vi "nanocal -- nuclear schottky fit V4.vi"() -> ()   [LabVIEW 2020] (continued)
\"τ1\"-> 0.024702194699  , \"τS\"-> 0.049753720072  , \"τN\"-> 0.002517387539  , \"τC\"-> 0.001542602546  , \"κ0\"-> 0.000000001719  , \"mm1\"-> 0.000000000000  , \"mm2\"-> 0.000000000000  , \"mm3\"-> 0.000000000000  , \"T\"->  0.308000000000  , \"B\"-> 5.000000000000  , \"θ\"-> 90.000000000000  |>   , \n\"IDS0340_210904_RAW_cal__sam_\" ->   <| \"ζ\"->  0.049152938826  , \"τ1\"-> 0.019216107215  , \"τS\"-> 0.064101941953  , \"τN\"-> 0.003869712687  , \"τC\"-> 0.002203680801  , \"κ0\"-> 0.000000001878  , \"mm1\"-> 0.000000000000  , \"mm2\"-> 0.000000000000  , \"mm3\"-> 0.000000000000  , \"T\"->  0.308000000000  , \"B\"-> 5.000000000000  , \"θ\"-> 90.000000000000  |>   , \n\"IDS0341_210904_RAW_cal__ref_\" ->   <| \"ζ\"->  0.059616809183  , \"τ1\"-> 0.023939570797  , \"τS\"-> 0.042653632086  , \"τN\"-> 0.001786288241  , \"τC\"-> 0.001975926031  , \"κ0\"-> 0.000000002092  , \"mm1\"-> 0.000000000000  , \"mm2\"-> 0.000000000000  , \"mm3\"-> 0.000000000000  , \"T\"->  0.360000000000  , \"B\"-> 5.000000000000  , \"θ\"-> 90.000000000000  |>   , \n\"IDS0341_210904_RAW_cal__sam_\" ->   <| \"ζ\"->  0.036041476168  , \"τ1\"-> 0.019203470752  , \"τS\"-> 0.054931014880  , \"τN\"-> 0.002271152158  , \"τC\"-> 0.002720100083  , \"κ0\"-> 0.000000002280  , \"mm1\"-> 0.000000000000  , \"mm2\"-> 0.000000000000  , \"mm3\"-> 0.000000000000  , \"T\"->  0.360000000000  , \"B\"-> 5.000000000000  , \"θ\"-> 90.000000000000  |>   , \n\"IDS0342_210904_RAW_cal__ref_\" ->   <| \"ζ\"->  0.044217232361  , \"τ1\"-> 0.023574215500  , \"τS\"-> 0.035981580515  , \"τN\"-> 0.001074333911  , \"τC\"-> 0.002351862552  , \"κ0\"-> 0.000000002629  , \"mm1\"-> 0.000000000000  , \"mm2\"-> 0.000000000000  , \"mm3\"-> 0.000000000000  , \"T\"->  0.438000000000  , \"B\"-> 5.000000000000  , \"θ\"-> 90.000000000000  |>   , \n\"IDS0342_210904_RAW_cal__sam_\" ->   <| \"ζ\"->  0.027360242550  , \"τ1\"-> 0.019369895135  , \"τS\"-> 0.046063450687  , \"τN\"-> 0.001549427641  , \"τC\"-> 0.003313507267  , \"κ0\"-> 0.000000002850  , \"mm1\"-> 0.000000000000  , \"mm2\"-> 0.000000000000  , \"mm3\"-> 0.000000000000  , \"T\"->  0.438000000000  , \"B\"-> 5.000000000000  , \"θ\"-> 90.000000000000  |>   , \n\"IDS0343_210904_RAW_cal__ref_\" ->   <| \"ζ\"->  0.035616644679  , \"τ1\"-> 0.021293989016  , \"τS\"-> 0.030504656314  , \"τN\"-> 0.000733387796  , \"τC\"-> 0.002756004742  , \"κ0\"-> 0.000000003268  , \"mm1\"-> 0.000000000000  , \"mm2\"-> 0.000000000000  , \"mm3\"-> 0.000000000000  , \"T\"->  0.530000000000  , \"B\"-> 5.000000000000  , \"θ\"-> 90.000000000000  |>   , \n\"IDS0343_210904_RAW_cal__sam_\" ->   <| \"ζ\"->  0.022691746072  , \"τ1\"-> 0.019361166937  , \"τS\"-> 0.038571137960  , \"τN\"-> 0.001037489181  , \"τC\"-> 0.004002961022  , \"κ0\"-> 0.000000003536  , \"mm1\"-> 0.000000000000  , \"mm2\"-> 0.000000000000  , \"mm3\"-> 0.000000000000  , \"T\"->  0.530000000000  , \"B\"-> 5.000000000000  , \"θ\"-> 90.000000000000  |>   , \n\"IDS0344_210904_RAW_cal__ref_\" ->   <| \"ζ\"->  0.029414072191  , \"τ1\"-> 0.022729389588  , \"τS\"-> 0.026807996891  , \"τN\"-> 0.000501873075  , \"τC\"-> 0.003020821681  , \"κ0\"-> 0.000000003880  , \"mm1\"-> 0.000000000000  , \"mm2\"-> 0.000000000000  , \"mm3\"-> 0.000000000000  , \"T\"->  0.620000000000  , \"B\"-> 5.000000000000  , \"θ\"-> 90.000000000000  |>   , \n\"IDS0344_210904_RAW_cal__sam_\" ->   <| \"ζ\"->  0.018598309928  , \"τ1\"-> 0.019376212159  , \"τS\"-> 0.033569863125  , \"τN\"-> 0.000771760425  , \"τC\"-> 0.004371934540  , \"κ0\"-> 0.000000004218  , \"mm1\"-> 0.000000000000  , \"mm2\"-> 0.000000000000  , \"mm3\"-> 0.000000000000  , \"T\"->  0.620000000000  , \"B\"-> 5.000000000000  , \"θ\"-> 90.000000000000  |>   , \n\"IDS0346_210904_RAW_cal__ref_\" ->   <| \"ζ\"->  0.351410523880  , \"τ1\"-> 0.038660935015  , \"τS\"-> 0.057750106762  , \"τN\"-> 0.192483765517  , \"τC\"-> 0.000883347451  , \"κ0\"-> 0.000000000403  , \"mm1\"-> 0.000000000000  , \"mm2\"-> 0.000000000000  , \"mm3\"-> 0.000000000000  , \"T\"->  0.122000000000  , \"B\"-> 8.000000000000  , \"θ\"-> 90.000000000000  |>   , \n\"IDS0346_210904_RAW_cal__sam_\" ->   <| \"ζ\"->  0.000000000000  , \"τ1\"-> 0.000000000000  , \"τS\"-> 0.000000000000  , \"τN\"-> 0.000000000000  , \"τC\"-> 0.000000000000  , \"κ0\"-> 0.000000000000  , \"mm1\"-> 0.000000000000  , \"mm2\"-> 0.000000000000  , \"mm3\"-> 0.000000000000  , \"T\"->  0.122000000000  , \"B\"-> 8.000000000000  , \"θ\"-> 90.000000000000  |>   , \n\"IDS0347_210906_RAW_cal__ref_\" ->   <| \"ζ\"->  0.282365663511  , \"τ1\"-> 0.039144945999  , \"τS\"-> 0.059953399264  , \"τN\"-> 0.108048405778  , \"τC\"-> 0.001096068963  , \"κ0\"-> 0.000000000641  , \"mm1\"-> 0.000000000000  , \"mm2\"-> 0.000000000000  , \"mm3\"-> 0.000000000000  , \"T\"->  0.157000000000  , \"B\"-> 8.000000000000  , \"θ\"-> 90.000000000000  |>   , \n\"IDS0347_210906_RAW_cal__sam_\" ->   <| \"ζ\"->  0.000000000000  , \"τ1\"-> 0.000000000000  , \"τS\"-> 0.000000000000  , \"τN\"-> 0.000000000000  , \"τC\"-> 0.000000000000  , \"κ0\"-> 0.000000000000  , \"mm1\"-> 0.000000000000  , \"mm2\"-> 0.000000000000  , \"mm3\"-> 0.000000000000  , \"T\"->  0.157000000000  , \"B\"-> 8.000000000000  , \"θ\"-> 90.000000000000  |>   , \n\"IDS0348_210906_RAW_cal__ref_\" ->   <| \"ζ\"->  0.231232733983  , \"τ1\"-> 0.036430431380  , \"τS\"-> 0.054781597050  , \"τN\"-> 0.064844477869  , \"τC\"-> 0.001068830966  , \"κ0\"-> 0.000000000760  , \"mm1\"-> 0.000000000000  , \"mm2\"-> 0.000000000000  , \"mm3\"-> 0.000000000000  , \"T\"->  0.178000000000  , \"B\"-> 8.000000000000  , \"θ\"-> 90.000000000000  |>   , \n\"IDS0348_210906_RAW_cal__sam_\" ->   <| \"ζ\"->  0.000000000000  , \"τ1\"-> 0.000000000000  , \"τS\"-> 0.000000000000  , \"τN\"-> 0.000000000000  , \"τC\"-> 0.000000000000  , \"κ0\"-> 0.000000000000  , \"mm1\"-> 0.000000000000  , \"mm2\"-> 0.000000000000  , \"mm3\"-> 0.000000000000  , \"T\"->  0.178000000000  , \"B\"-> 8.000000000000  , \"θ\"-> 90.000000000000  |>   , \n\"IDS0349_210906_RAW_cal__ref_\" ->   <| \"ζ\"->  0.190485473901  , \"τ1\"-> 0.032323616024  , \"τS\"-> 0.052823523941  , \"τN\"-> 0.036537332757  , \"τC\"-> 0.001181014846  , \"κ0\"-> 0.000000001037  , \"mm1\"-> 0.000000000000  , \"mm2\"-> 0.000000000000  , \"mm3\"-> 0.000000000000  , \"T\"->  0.200000000000  , \"B\"-> 8.000000000000  , \"θ\"-> 90.000000000000  |>   , \n\"IDS0349_210906_RAW_cal__sam_\" ->   <| \"ζ\"->  0.000000000000  , \"τ1\"-> 0.000000000000  , \"τS\"-> 0.000000000000  , \"τN\"-> 0.000000000000  , \"τC\"-> 0.000000000000  , \"κ0\"-> 0.000000000000  , \"mm1\"-> 0.000000000000  , \"mm2\"-> 0.000000000000  , \"mm3\"-> 0.000000000000  , \"T\"->  0.200000000000  , \"B\"-> 8.000000000000  , \"θ\"-> 90.000000000000  |>   , \n\"IDS0350_210906_RAW_cal__ref_\" ->   <| \"ζ\"->  0.118733755426  , \"τ1\"-> 0.027090622935  , \"τS\"-> 0.042154952610  , \"τN\"-> 0.016299612233  , \"τC\"-> 0.001268322773  , \"κ0\"-> 0.000000001347  , \"mm1\"-> 0.000000000000  , \"mm2\"-> 0.000000000000  , \"mm3\"-> 0.000000000000  , \"T\"->  0.260000000000  , \"B\"-> 8.000000000000  , \"θ\"-> 90.000000000000  |>   , \n\"IDS0350_210906_RAW_cal__sam_\" ->   <| \"ζ\"->  0.000000000000  , \"τ1\"-> 0.000000000000  , \"τS\"-> 0.000000000000  , \"τN\"-> 0.000000000000  , \"τC\"-> 0.000000000000  , \"κ0\"-> 0.000000000000  , \"mm1\"-> 0.000000000000  , \"mm2\"-> 0.000000000000  , \"mm3\"-> 0.000000000000  , \"T\"->  0.260000000000  , \"B\"-> 8.000000000000  , \"θ\"-> 90.000000000000  |>   , \n\"IDS0351_210906_RAW_cal__ref_\" ->   <| \"ζ\"->  0.081031099964  , \"τ1\"-> 0.021876847581  , \"τS\"-> 0.037173038366  , \"τN\"-> 0.007845971856  , \"τC\"-> 0.001561862252  , \"κ0\"-> 0.000000001761  , \"mm1\"-> 0.000000000000  , \"mm2\"-> 0.000000000000  , \"mm3\"-> 0.000000000000  , \"T\"->  0.310000000000  , \"B\"-> 8.000000000000  , \"θ\"-> 90.000000000000  |>   , \n\"IDS0351_210906_RAW_cal__sam_\" ->   <| \"ζ\"->  0.000000000000  , \"τ1\"-> 0.000000000000  , \"τS\"-> 0.000000000000  , \"τN\"-> 0.000000000000  , \"τC\"-> 0.000000000000  , \"κ0\"-> 0.000000000000  , \"mm1\"-> 0.000000000000  , \"mm2\"-> 0.000000000000  , \"mm3\"-> 0.000000000000  , \"T\"->  0.310000000000  , \"B\"-> 8.000000000000  , \"θ\"-> 90.000000000000  |>   , \n\"IDS0352_210906_RAW_cal__ref_\" ->   <| \"ζ\"->  0.060336863550  , \"τ1\"-> 0.020607625563  , \"τS\"-> 0.034334079822  , \"τN\"-> 0.004923011954  , \"τC\"-> 0.001895452704  , \"κ0\"-> 0.000000002106  , \"mm1\"-> 0.000000000000  , \"mm2\"-> 0.000000000000  , \"mm3\"-> 0.000000000000  , \"T\"->  0.360000000000  , \"B\"-> 8.000000000000  , \"θ\"-> 90.000000000000  |>   , \n\"IDS0352_210906_RAW_cal__sam_\" ->   <| \"ζ\"->  0.000000000000  , \"τ1\"-> 0.000000000000  , \"τS\"-> 0.000000000000  , \"τN\"-> 0.000000000000  , \"τC\"-> 0.000000000000  , \"κ0\"-> 0.000000000000  , \"mm1\"-> 0.000000000000  , \"mm2\"-> 0.000000000000  , \"mm3\"-> 0.000000000000  , \"T\"->  0.360000000000  , \"B\"-> 8.000000000000  , \"θ\"-> 90.000000000000  |>   , \n\"IDS0353_210906_RAW_cal__ref_\" ->   <| \"ζ\"->  0.045012118583  , \"τ1\"-> 0.020623291685  , \"τS\"-> 0.031197986163  , \"τN\"-> 0.002724775132  , \"τC\"-> 0.002225741907  , \"κ0\"-> 0.000000002626  , \"mm1\"-> 0.000000000000  , \"mm2\"-> 0.000000000000  , \"mm3\"-> 0.000000000000  , \"T\"->  0.438000000000  , \"B\"-> 8.000000000000  , \"θ\"-> 90.000000000000  |>   , \n\"IDS0353_210906_RAW_cal__sam_\" ->   <| \"ζ\"->  0.000000000000  , \"τ1\"-> 0.000000000000  , \"τS\"-> 0.000000000000  , \"τN\"-> 0.000000000000  , \"τC\"-> 0.000000000000  , \"κ0\"-> 0.000000000000  , \"mm1\"-> 0.000000000000  , \"mm2\"-> 0.000000000000  , \"mm3\"-> 0.000000000000  , \"T\"->  0.438000000000  , \"B\"-> 8.000000000000  , \"θ\"-> 90.000000000000  |>   , \n\"IDS0354_210906_RAW_cal__ref_\" ->   <| \"ζ\"->  0.035878229865  , \"τ1\"-> 0.020618191238  , \"τS\"-> 0.028341492437  , \"τN\"-> 0.001542437572  , \"τC\"-> 0.002465046672  , \"κ0\"-> 0.000000003272  , \"mm1\"-> 0.000000000000  , \"mm2\"-> 0.000000000000  , \"mm3\"-> 0.000000000000  , \"T\"->  0.530000000000  , \"B\"-> 8.000000000000  , \"θ\"-> 90.000000000000  |>   , \n\"IDS0354_210906_RAW_cal__sam_\" ->   <| \"ζ\"->  0.000000000000  , \"τ1\"-> 0.000000000000  , \"τS\"-> 0.000000000000  , \"τN\"-> 0.000000000000  , \"τC\"-> 0.000000000000  , \"κ0\"-> 0.000000000000  , \"mm1\"-> 0.000000000000  , \"mm2\"-> 0.000000000000  , \"mm3\"-> 0.000000000000  , \"T\"->  0.530000000000  , \"B\"-> 8.000000000000  , \"θ\"-> 90.000000000000  |>   , \n\"IDS0355_210906_RAW_cal__ref_\" ->   <| \"ζ\"->  0.022259133140  , \"τ1\"-> 0.021062021806  , \"τS\"-> 0.021361272182  , \"τN\"-> 0.000526217477  , \"τC\"-> 0.003770290408  , \"κ0\"-> 0.000000005411  , \"mm1\"-> 0.000000000000  , \"mm2\"-> 0.000000000000  , \"mm3\"-> 0.000000000000  , \"T\"->  0.830000000000  , \"B\"-> 8.000000000000  , \"θ\"-> 90.000000000000  |>   , \n\"IDS0355_210906_RAW_cal__sam_\" ->   <| \"ζ\"->  0.000000000000  , \"τ1\"-> 0.000000000000  , \"τS\"-> 0.000000000000  , \"τN\"-> 0.000000000000  , \"τC\"-> 0.000000000000  , \"κ0\"-> 0.000000000000  , \"mm1\"-> 0.000000000000  , \"mm2\"-> 0.000000000000  , \"mm3\"-> 0.000000000000  , \"T\"->  0.830000000000  , \"B\"-> 8.000000000000  , \"θ\"-> 90.000000000000  |>   , \n\"IDS0359_210907_RAW_cal__ref_\" ->   <| \"ζ\"->  0.381003010305  , \"τ1\"-> 0.083336505244  , \"τS\"-> 0.050211621127  , \"τN\"-> 0.550745531665  , \"τC\"-> 0.000692694606  , \"κ0\"-> 0.000000000382  , \"mm1\"-> 0.000000000000  , \"mm2\"-> 0.000000000000  , \"mm3\"-> 0.000000000000  , \"T\"->  0.120000000000  , \"B\"-> 12.000000000000  , \"θ\"-> 60.000000000000  |>   , \n\"IDS0359_210907_RAW_cal__sam_\" ->   <| \"ζ\"->  0.000000000000  , \"τ1\"-> 0.000000000000  , \"τS\"-> 0.000000000000  , \"τN\"-> 0.000000000000  , \"τC\"-> 0.000000000000  , \"κ0\"-> 0.000000000000  , \"mm1\"-> 0.000000000000  , \"mm2\"-> 0.000000000000  , \"mm3\"-> 0.000000000000  , \"T\"->  0.120000000000  , \"B\"-> 12.000000000000  , \"θ\"-> 60.000000000000  |>   , \n\"IDS0360_210907_RAW_cal__ref_\" ->   <| \"ζ\"->  0.323840637004  , \"τ1\"-> 0.072581646931  , \"τS\"-> 0.047951414335  , \"τN\"-> 0.283785405218  , \"τC\"-> 0.000913184933  , \"κ0\"-> 0.000000000636  , \"mm1\"-> 0.000000000000  , \"mm2\"-> 0.000000000000  , \"mm3\"-> 0.000000000000  , \"T\"->  0.150000000000  , \"B\"-> 12.000000000000  , \"θ\"-> 60.000000000000  |>   , \n\"IDS0360_210907_RAW_cal__sam_\" ->   <| \"ζ\"->  0.000000000000  , \"τ1\"-> 0.000000000000  , \"τS\"-> 0.000000000000  , \"τN\"-> 0.000000000000  , \"τC\"-> 0.000000000000  , \"κ0\"-> 0.000000000000  , \"mm1\"-> 0.000000000000  , \"mm2\"-> 0.000000000000  , \"mm3\"-> 0.000000000000  , \"T\"->  0.150000000000  , \"B\"-> 12.000000000000  , \"θ\"-> 60.000000000000  |>   , \n\"IDS0361_210908_RAW_cal__ref_\" ->   <| \"ζ\"->  0.279940228007  , \"τ1\"-> 0.067057240536  , \"τS\"-> 0.048025817643  , \"τN\"-> 0.170011495172  , \"τC\"-> 0.001015047914  , \"κ0\"-> 0.000000000754  , \"mm1\"-> 0.000000000000  , \"mm2\"-> 0.000000000000  , \"mm3\"-> 0.000000000000  , \"T\"->  0.168000000000  , \"B\"-> 12.000000000000  , \"θ\"-> 60.000000000000  |>   , \n\"IDS0361_210908_RAW_cal__sam_\" ->   <| \"ζ\"->  0.000000000000  , \"τ1\"-> 0.000000000000  , \"τS\"-> 0.000000000000  , \"τN\"-> 0.000000000000  , \"τC\"-> 0.000000000000  , \"κ0\"-> 0.000000000000  , \"mm1\"-> 0.000000000000  , \"mm2\"-> 0.000000000000  , \"mm3\"-> 0.000000000000  , \"T\"->  0.168000000000  , \"B\"-> 12.000000000000  , \"θ\"-> 60.000000000000  |>   , \n\"IDS0362_210908_RAW_cal__ref_\" ->   <| \"ζ\"->  0.206594976212  , \"τ1\"-> 0.057885925979  , \"τS\"-> 0.038698575169  , \"τN\"-> 0.092347634602  , \"τC\"-> 0.001108131545  , \"κ0\"-> 0.000000001046  , \"mm1\"-> 0.000000000000  , \"mm2\"-> 0.000000000000  , \"mm3\"-> 0.000000000000  , \"T\"->  0.197000000000  , \"B\"-> 12.000000000000  , \"θ\"-> 60.000000000000  |>   , \n\"IDS0362_210908_RAW_cal__sam_\" ->   <| \"ζ\"->  0.000000000000  , \"τ1\"-> 0.000000000000  , \"τS\"-> 0.000000000000  , \"τN\"-> 0.000000000000  , \"τC\"-> 0.000000000000  , \"κ0\"-> 0.000000000000  , \"mm1\"-> 0.000000000000  , \"mm2\"-> 0.000000000000  , \"mm3\"-> 0.000000000000  , \"T\"->  0.197000000000  , \"B\"-> 12.000000000000  , \"θ\"-> 60.000000000000  |>   , \n\"IDS0363_210908_RAW_cal__ref_\" ->   <| \"ζ\"->  0.123216898961  , \"τ1\"-> 0.041424716624  , \"τS\"-> 0.030606562009  , \"τN\"-> 0.033679175657  , \"τC\"-> 0.001245281919  , \"κ0\"-> 0.000000001353  , \"mm1\"-> 0.000000000000  , \"mm2\"-> 0.000000000000  , \"mm3\"-> 0.000000000000  , \"T\"->  0.250000000000  , \"B\"-> 12.000000000000  , \"θ\"-> 60.000000000000  |>   , \n\"IDS0363_210908_RAW_cal__sam_\" ->   <| \"ζ\"->  0.000000000000  , \"τ1\"-> 0.000000000000  , \"τS\"-> 0.000000000000  , \"τN\"-> 0.000000000000  , \"τC\"-> 0.000000000000  , \"κ0\"-> 0.000000000000  , \"mm1\"-> 0.000000000000  , \"mm2\"-> 0.000000000000  , \"mm3\"-> 0.000000000000  , \"T\"->  0.250000000000  , \"B\"-> 12.000000000000  , \"θ\"-> 60.000000000000  |>   , \n\"IDS0364_210908_RAW_cal__ref_\" ->   <| \"ζ\"->  0.083979493288  , \"τ1\"-> 0.035863468022  , \"τS\"-> 0.027413945050  , \"τN\"-> 0.017174500536  , \"τC\"-> 0.001551957186  , \"κ0\"-> 0.000000001738  , \"mm1\"-> 0.000000000000  , \"mm2\"-> 0.000000000000  , \"mm3\"-> 0.000000000000  , \"T\"->  0.307000000000  , \"B\"-> 12.000000000000  , \"θ\"-> 60.000000000000  |>   , \n\"IDS0364_210908_RAW_cal__sam_\" ->   <| \"ζ\"->  0.000000000000  , \"τ1\"-> 0.000000000000  , \"τS\"-> 0.000000000000  , \"τN\"-> 0.000000000000  , \"τC\"-> 0.000000000000  , \"κ0\"-> 0.000000000000  , \"mm1\"-> 0.000000000000  , \"mm2\"-> 0.000000000000  , \"mm3\"-> 0.000000000000  , \"T\"->  0.307000000000  , \"B\"-> 12.000000000000  , \"θ\"-> 60.000000000000  |>   , \n\"IDS0365_210908_RAW_cal__ref_\" ->   <| \"ζ\"->  0.061526991224  , \"τ1\"-> 0.029624261727  , \"τS\"-> 0.025208021627  , \"τN\"-> 0.009698502183  , \"τC\"-> 0.001918212332  , \"κ0\"-> 0.000000002116  , \"mm1\"-> 0.000000000000  , \"mm2\"-> 0.000000000000  , \"mm3\"-> 0.000000000000  , \"T\"->  0.360000000000  , \"B\"-> 12.000000000000  , \"θ\"-> 60.000000000000  |>   , \n\"IDS0365_210908_RAW_cal__sam_\" ->   <| \"ζ\"->  0.000000000000  , \"τ1\"-> 0.000000000000  , \"τS\"-> 0.000000000000  , \"τN\"-> 0.000000000000  , \"τC\"-> 0.000000000000  , \"κ0\"-> 0.000000000000  , \"mm1\"-> 0.000000000000  , \"mm2\"-> 0.000000000000  , \"mm3\"-> 0.000000000000  , \"T\"->  0.360000000000  , \"B\"-> 12.000000000000  , \"θ\"-> 60.000000000000  |>   , \n\"IDS0366_210908_RAW_cal__ref_\" ->   <| \"ζ\"->  0.045515267447  , \"τ1\"-> 0.026001810196  , \"τS\"-> 0.023136668780  , \"τN\"-> 0.005224117981  , \"τC\"-> 0.002327400857  , \"κ0\"-> 0.000000002646  , \"mm1\"-> 0.000000000000  , \"mm2\"-> 0.000000000000  , \"mm3\"-> 0.000000000000  , \"T\"->  0.430000000000  , \"B\"-> 12.000000000000  , \"θ\"-> 60.000000000000  |>   , \n\"IDS0366_210908_RAW_cal__sam_\" ->   <| \"ζ\"->  0.000000000000  , \"τ1\"-> 0.000000000000  , \"τS\"-> 0.000000000000  , \"τN\"-> 0.000000000000  , \"τC\"-> 0.000000000000  , \"κ0\"-> 0.000000000000  , \"mm1\"-> 0.000000000000  , \"mm2\"-> 0.000000000000  , \"mm3\"-> 0.000000000000  , \"T\"->  0.430000000000  , \"B\"-> 12.000000000000  , \"θ\"-> 60.000000000000  |>   , \n\"IDS0367_210908_RAW_cal__ref_\" ->   <| \"ζ\"->  0.037324451442  , \"τ1\"-> 0.019605264024  , \"τS\"-> 0.021700560504  , \"τN\"-> 0.002800944156  , \"τC\"-> 0.002526998509  , \"κ0\"-> 0.000000003301  , \"mm1\"-> 0.000000000000  , \"mm2\"-> 0.000000000000  , \"mm3\"-> 0.000000000000  , \"T\"->  0.530000000000  , \"B\"-> 12.000000000000  , \"θ\"-> 60.000000000000  |>   , \n\"IDS0367_210908_RAW_cal__sam_\" ->   <| \"ζ\"->  0.000000000000  , \"τ1\"-> 0.000000000000  , \"τS\"-> 0.000000000000  , \"τN\"-> 0.000000000000  , \"τC\"-> 0.000000000000  , \"κ0\"-> 0.000000000000  , \"mm1\"-> 0.000000000000  , \"mm2\"-> 0.000000000000  , \"mm3\"-> 0.000000000000  , \"T\"->  0.530000000000  , \"B\"-> 12.000000000000  , \"θ\"-> 60.000000000000  |>   , \n\"IDS0368_210908_RAW_cal__ref_\" ->   <| \"ζ\"->  0.030581023885  , \"τ1\"-> 0.017326525290  , \"τS\"-> 0.020225378130  , \"τN\"-> 0.001703135365  , \"τC\"-> 0.003380889395  , \"κ0\"-> 0.000000003914  , \"mm1\"-> 0.000000000000  , \"mm2\"-> 0.000000000000  , \"mm3\"-> 0.000000000000  , \"T\"->  0.630000000000  , \"B\"-> 12.000000000000  , \"θ\"-> 60.000000000000  |>   , \n\"IDS0368_210908_RAW_cal__sam_\" ->   <| \"ζ\"->  0.000000000000  , \"τ1\"-> 0.000000000000  , \"τS\"-> 0.000000000000  , \"τN\"-> 0.000000000000  , \"τC\"-> 0.000000000000  , \"κ0\"-> 0.000000000000  , \"mm1\"-> 0.000000000000  , \"mm2\"-> 0.000000000000  , \"mm3\"-> 0.000000000000  , \"T\"->  0.630000000000  , \"B\"-> 12.000000000000  , \"θ\"-> 60.000000000000  |>   , \n\"IDS0369_210908_RAW_cal__ref_\" ->   <| \"ζ\"->  0.022212344829  , \"τ1\"-> 0.017343641344  , \"τS\"-> 0.018001662092  , \"τN\"-> 0.000711569404  , \"τC\"-> 0.004309595418  , \"κ0\"-> 0.000000005439  , \"mm1\"-> 0.000000000000  , \"mm2\"-> 0.000000000000  , \"mm3\"-> 0.000000000000  , \"T\"->  0.830000000000  , \"B\"-> 12.000000000000  , \"θ\"-> 60.000000000000  |>   , \n\"IDS0369_210908_RAW_cal__sam_\" ->   <| \"ζ\"->  0.000000000000  , \"τ1\"-> 0.000000000000  , \"τS\"-> 0.000000000000  , \"τN\"-> 0.000000000000  , \"τC\"-> 0.000000000000  , \"κ0\"-> 0.000000000000  , \"mm1\"-> 0.000000000000  , \"mm2\"-> 0.000000000000  , \"mm3\"-> 0.000000000000  , \"T\"->  0.830000000000  , \"B\"-> 12.000000000000  , \"θ\"-> 60.000000000000  |>   , \n\"IDS0370_210908_RAW_cal__ref_\" ->   <| \"ζ\"->  0.021569402950  , \"τ1\"-> 0.017921737944  , \"τS\"-> 0.015463128015  , \"τN\"-> 0.000390873619  , \"τC\"-> 0.004954240411  , \"κ0\"-> 0.000000007586  , \"mm1\"-> 0.000000000000  , \"mm2\"-> 0.000000000000  , \"mm3\"-> 0.000000000000  , \"T\"->  1.130000000000  , \"B\"-> 12.000000000000  , \"θ\"-> 60.000000000000  |>   , \n\"IDS0370_210908_RAW_cal__sam_\" ->   <| \"ζ\"->  0.000000000000  , \"τ1\"-> 0.000000000000  , \"τS\"-> 0.000000000000  , \"τN\"-> 0.000000000000  , \"τC\"-> 0.000000000000  , \"κ0\"-> 0.000000000000  , \"mm1\"-> 0.000000000000  , \"mm2\"-> 0.000000000000  , \"mm3\"-> 0.000000000000  , \"T\"->  1.130000000000  , \"B\"-> 12.000000000000  , \"θ\"-> 60.000000000000  |>   , \n\"IDS0371_210908_RAW_cal__ref_\" ->   <| \"ζ\"->  0.020664849580  , \"τ1\"-> 0.018108723176  , \"τS\"-> 0.010299896170  , \"τN\"-> 0.000079818017  , \"τC\"-> 0.006259144045  , \"κ0\"-> 0.000000013130  , \"mm1\"-> 0.000000000000  , \"mm2\"-> 0.000000000000  , \"mm3\"-> 0.000000000000  , \"T\"->  1.900000000000  , \"B\"-> 12.000000000000  , \"θ\"-> 60.000000000000  |>   , \n\"IDS0371_210908_RAW_cal__sam_\" ->   <| \"ζ\"->  0.000000000000  , \"τ1\"-> 0.000000000000  , \"τS\"-> 0.000000000000  , \"τN\"-> 0.000000000000  , \"τC\"-> 0.000000000000  , \"κ0\"-> 0.000000000000  , \"mm1\"-> 0.000000000000  , \"mm2\"-> 0.000000000000  , \"mm3\"-> 0.000000000000  , \"T\"->  1.900000000000  , \"B\"-> 12.000000000000  , \"θ\"-> 60.000000000000  |>   , \n\"IDS0372_210908_RAW_cal__ref_\" ->   <| \"ζ\"->  0.021592146431  , \"τ1\"-> 0.018093446545  , \"τS\"-> 0.007071841556  , \"τN\"-> 0.000029085223  , \"τC\"-> 0.005341206531  , \"κ0\"-> 0.000000023517  , \"mm1\"-> 0.000000000000  , \"mm2\"-> 0.000000000000  , \"mm3\"-> 0.000000000000  , \"T\"->  3.110000000000  , \"B\"-> 12.000000000000  , \"θ\"-> 60.000000000000  |>   , \n\"IDS0372_210908_RAW_cal__sam_\" ->   <| \"ζ\"->  0.000000000000  , \"τ1\"-> 0.000000000000  , \"τS\"-> 0.000000000000  , \"τN\"-> 0.000000000000  , \"τC\"-> 0.000000000000  , \"κ0\"-> 0.000000000000  , \"mm1\"-> 0.000000000000  , \"mm2\"-> 0.000000000000  , \"mm3\"-> 0.000000000000  , \"T\"->  3.110000000000  , \"B\"-> 12.000000000000  , \"θ\"-> 60.000000000000  |>   , \n\"IDS0373_210908_RAW_cal__ref_\" ->   <| \"ζ\"->  0.028148688120  , \"τ1\"-> 0.012706961955  , \"τS\"-> 0.003881518121  , \"τN\"-> 0.000007160132  , \"τC\"-> 0.004346615253  , \"κ0\"-> 0.000000058313  , \"mm1\"-> 0.000000000000  , \"mm2\"-> 0.000000000000  , \"mm3\"-> 0.000000000000  , \"T\"->  5.750000000000  , \"B\"-> 12.000000000000  , \"θ\"-> 60.000000000000  |>   , \n\"IDS0373_210908_RAW_cal__sam_\" ->   <| \"ζ\"->  0.000000000000  , \"τ1\"-> 0.000000000000  , \"τS\"-> 0.000000000000  , \"τN\"-> 0.000000000000  , \"τC\"-> 0.000000000000  , \"κ0\"-> 0.000000000000  , \"mm1\"-> 0.000000000000  , \"mm2\"-> 0.000000000000  , \"mm3\"-> 0.000000000000  , \"T\"->  5.750000000000  , \"B\"-> 12.000000000000  , \"θ\"-> 60.000000000000  |>   , \n\"IDS0377_210909_RAW_cal__ref_\" ->   <| \"ζ\"->  0.217996441376  , \"τ1\"-> 0.079837328848  , \"τS\"-> 0.035140385542  , \"τN\"-> 0.027062270101  , \"τC\"-> 0.001091238478  , \"κ0\"-> 0.000000001044  , \"mm1\"-> 0.000000000000  , \"mm2\"-> 0.000000000000  , \"mm3\"-> 0.000000000000  , \"T\"->  0.197000000000  , \"B\"-> 8.000000000000  , \"θ\"-> 0.000000000000  |>   , \n\"IDS0377_210909_RAW_cal__sam_\" ->   <| \"ζ\"->  0.132375437908  , \"τ1\"-> 0.085614291193  , \"τS\"-> 0.046888304266  , \"τN\"-> 0.035744833495  , \"τC\"-> 0.001504622490  , \"κ0\"-> 0.000000001156  , \"mm1\"-> 0.000000000000  , \"mm2\"-> 0.000000000000  , \"mm3\"-> 0.000000000000  , \"T\"->  0.197000000000  , \"B\"-> 8.000000000000  , \"θ\"-> 0.000000000000  |>   , \n\"IDS0378_210909_RAW_cal__ref_\" ->   <| \"ζ\"->  0.444097524539  , \"τ1\"-> 0.128858676931  , \"τS\"-> 0.109017650637  , \"τN\"-> 0.152310736136  , \"τC\"-> 0.001225116605  , \"κ0\"-> 0.000000000395  , \"mm1\"-> 0.000000000000  , \"mm2\"-> 0.000000000000  , \"mm3\"-> 0.000000000000  , \"T\"->  0.122000000000  , \"B\"-> 8.000000000000  , \"θ\"-> 0.000000000000  |>   , \n\"IDS0378_210909_RAW_cal__sam_\" ->   <| \"ζ\"->  0.278068103221  , \"τ1\"-> 0.118058810167  , \"τS\"-> 0.149294349958  , \"τN\"-> 0.128211590058  , \"τC\"-> 0.001553934408  , \"κ0\"-> 0.000000000522  , \"mm1\"-> 0.000000000000  , \"mm2\"-> 0.000000000000  , \"mm3\"-> 0.000000000000  , \"T\"->  0.122000000000  , \"B\"-> 8.000000000000  , \"θ\"-> 0.000000000000  |>   , \n\"IDS0379_210909_RAW_cal__ref_\" ->   <| \"ζ\"->  0.358674724692  , \"τ1\"-> 0.106557394659  , \"τS\"-> 0.062757387956  , \"τN\"-> 0.083491977845  , \"τC\"-> 0.001111110425  , \"κ0\"-> 0.000000000629  , \"mm1\"-> 0.000000000000  , \"mm2\"-> 0.000000000000  , \"mm3\"-> 0.000000000000  , \"T\"->  0.148000000000  , \"B\"-> 8.000000000000  , \"θ\"-> 0.000000000000  |>   , \n\"IDS0379_210909_RAW_cal__sam_\" ->   <| \"ζ\"->  0.225754480330  , \"τ1\"-> 0.098523892400  , \"τS\"-> 0.080528394696  , \"τN\"-> 0.096491011881  , \"τC\"-> 0.001394999535  , \"κ0\"-> 0.000000000751  , \"mm1\"-> 0.000000000000  , \"mm2\"-> 0.000000000000  , \"mm3\"-> 0.000000000000  , \"T\"->  0.148000000000  , \"B\"-> 8.000000000000  , \"θ\"-> 0.000000000000  |>   , \n\"IDS0380_210909_RAW_cal__ref_\" ->   <| \"ζ\"->  0.289033994940  , \"τ1\"-> 0.085284172773  , \"τS\"-> 0.050519531224  , \"τN\"-> 0.055850802998  , \"τC\"-> 0.001015487958  , \"κ0\"-> 0.000000000740  , \"mm1\"-> 0.000000000000  , \"mm2\"-> 0.000000000000  , \"mm3\"-> 0.000000000000  , \"T\"->  0.168000000000  , \"B\"-> 8.000000000000  , \"θ\"-> 0.000000000000  |>   , \n\"IDS0380_210909_RAW_cal__sam_\" ->   <| \"ζ\"->  0.175421092430  , \"τ1\"-> 0.089198304544  , \"τS\"-> 0.059713999657  , \"τN\"-> 0.066015553792  , \"τC\"-> 0.001291009219  , \"κ0\"-> 0.000000000858  , \"mm1\"-> 0.000000000000  , \"mm2\"-> 0.000000000000  , \"mm3\"-> 0.000000000000  , \"T\"->  0.168000000000  , \"B\"-> 8.000000000000  , \"θ\"-> 0.000000000000  |>   , \n\"IDS0381_210909_RAW_cal__ref_\" ->   <| \"ζ\"->  0.126932147164  , \"τ1\"-> 0.058068643235  , \"τS\"-> 0.026925290066  , \"τN\"-> 0.010981117446  , \"τC\"-> 0.001219952265  , \"κ0\"-> 0.000000001350  , \"mm1\"-> 0.000000000000  , \"mm2\"-> 0.000000000000  , \"mm3\"-> 0.000000000000  , \"T\"->  0.250000000000  , \"B\"-> 8.000000000000  , \"θ\"-> 0.000000000000  |>   , \n\"IDS0381_210909_RAW_cal__sam_\" ->   <| \"ζ\"->  0.078113399712  , \"τ1\"-> 0.055920008457  , \"τS\"-> 0.035460304856  , \"τN\"-> 0.012612271055  , \"τC\"-> 0.001663430483  , \"κ0\"-> 0.000000001497  , \"mm1\"-> 0.000000000000  , \"mm2\"-> 0.000000000000  , \"mm3\"-> 0.000000000000  , \"T\"->  0.250000000000  , \"B\"-> 8.000000000000  , \"θ\"-> 0.000000000000  |>   , \n\"IDS0382_210909_RAW_cal__ref_\" ->   <| \"ζ\"->  0.087249653273  , \"τ1\"-> 0.047168507247  , \"τS\"-> 0.024336865487  , \"τN\"-> 0.005605961335  , \"τC\"-> 0.001526895316  , \"κ0\"-> 0.000000001730  , \"mm1\"-> 0.000000000000  , \"mm2\"-> 0.000000000000  , \"mm3\"-> 0.000000000000  , \"T\"->  0.300000000000  , \"B\"-> 8.000000000000  , \"θ\"-> 0.000000000000  |>   , \n\"IDS0382_210909_RAW_cal__sam_\" ->   <| \"ζ\"->  0.054029770351  , \"τ1\"-> 0.051440847518  , \"τS\"-> 0.032079834642  , \"τN\"-> 0.007150632998  , \"τC\"-> 0.002202148776  , \"κ0\"-> 0.000000001884  , \"mm1\"-> 0.000000000000  , \"mm2\"-> 0.000000000000  , \"mm3\"-> 0.000000000000  , \"T\"->  0.300000000000  , \"B\"-> 8.000000000000  , \"θ\"-> 0.000000000000  |>   , \n\"IDS0383_210910_RAW_cal__ref_\" ->   <| \"ζ\"->  0.062586766538  , \"τ1\"-> 0.048322657274  , \"τS\"-> 0.023582446152  , \"τN\"-> 0.003596780616  , \"τC\"-> 0.001965770478  , \"κ0\"-> 0.000000002106  , \"mm1\"-> 0.000000000000  , \"mm2\"-> 0.000000000000  , \"mm3\"-> 0.000000000000  , \"T\"->  0.360000000000  , \"B\"-> 8.000000000000  , \"θ\"-> 0.000000000000  |>   , \n\"IDS0383_210910_RAW_cal__sam_\" ->   <| \"ζ\"->  0.038341835326  , \"τ1\"-> 0.050866858713  , \"τS\"-> 0.030652081909  , \"τN\"-> 0.004623805952  , \"τC\"-> 0.002823684758  , \"κ0\"-> 0.000000002289  , \"mm1\"-> 0.000000000000  , \"mm2\"-> 0.000000000000  , \"mm3\"-> 0.000000000000  , \"T\"->  0.360000000000  , \"B\"-> 8.000000000000  , \"θ\"-> 0.000000000000  |>   , \n\"IDS0384_210910_RAW_cal__ref_\" ->   <| \"ζ\"->  0.047320664202  , \"τ1\"-> 0.050730770684  , \"τS\"-> 0.023716512211  , \"τN\"-> 0.002200072160  , \"τC\"-> 0.002249629457  , \"κ0\"-> 0.000000002636  , \"mm1\"-> 0.000000000000  , \"mm2\"-> 0.000000000000  , \"mm3\"-> 0.000000000000  , \"T\"->  0.430000000000  , \"B\"-> 8.000000000000  , \"θ\"-> 0.000000000000  |>   , \n\"IDS0384_210910_RAW_cal__sam_\" ->   <| \"ζ\"->  0.029950572027  , \"τ1\"-> 0.044923259835  , \"τS\"-> 0.030416367718  , \"τN\"-> 0.002541256331  , \"τC\"-> 0.003331031560  , \"κ0\"-> 0.000000002858  , \"mm1\"-> 0.000000000000  , \"mm2\"-> 0.000000000000  , \"mm3\"-> 0.000000000000  , \"T\"->  0.430000000000  , \"B\"-> 8.000000000000  , \"θ\"-> 0.000000000000  |>   , \n\"IDS0385_210910_RAW_cal__ref_\" ->   <| \"ζ\"->  0.037147896010  , \"τ1\"-> 0.047226564206  , \"τS\"-> 0.024619467421  , \"τN\"-> 0.001310789285  , \"τC\"-> 0.002565709752  , \"κ0\"-> 0.000000003275  , \"mm1\"-> 0.000000000000  , \"mm2\"-> 0.000000000000  , \"mm3\"-> 0.000000000000  , \"T\"->  0.530000000000  , \"B\"-> 8.000000000000  , \"θ\"-> 0.000000000000  |>   , \n\"IDS0385_210910_RAW_cal__sam_\" ->   <| \"ζ\"->  0.024600756648  , \"τ1\"-> 0.043958236582  , \"τS\"-> 0.031312750224  , \"τN\"-> 0.001348105931  , \"τC\"-> 0.003635120795  , \"κ0\"-> 0.000000003548  , \"mm1\"-> 0.000000000000  , \"mm2\"-> 0.000000000000  , \"mm3\"-> 0.000000000000  , \"T\"->  0.530000000000  , \"B\"-> 8.000000000000  , \"θ\"-> 0.000000000000  |>   , \n\"IDS0386_210910_RAW_cal__ref_\" ->   <| \"ζ\"->  0.028995432115  , \"τ1\"-> 0.046559455187  , \"τS\"-> 0.026126949833  , \"τN\"-> 0.000676599034  , \"τC\"-> 0.003300199116  , \"κ0\"-> 0.000000003897  , \"mm1\"-> 0.000000000000  , \"mm2\"-> 0.000000000000  , \"mm3\"-> 0.000000000000  , \"T\"->  0.630000000000  , \"B\"-> 8.000000000000  , \"θ\"-> 0.000000000000  |>   , \n\"IDS0386_210910_RAW_cal__sam_\" ->   <| \"ζ\"->  0.019494767421  , \"τ1\"-> 0.040349410363  , \"τS\"-> 0.033202805363  , \"τN\"-> 0.000770756985  , \"τC\"-> 0.004303152006  , \"κ0\"-> 0.000000004241  , \"mm1\"-> 0.000000000000  , \"mm2\"-> 0.000000000000  , \"mm3\"-> 0.000000000000  , \"T\"->  0.630000000000  , \"B\"-> 8.000000000000  , \"θ\"-> 0.000000000000  |>   , \n\"IDS0387_210910_RAW_cal__ref_\" ->   <| \"ζ\"->  0.021158107821  , \"τ1\"-> 0.047181877660  , \"τS\"-> 0.030519366684  , \"τN\"-> 0.000257878410  , \"τC\"-> 0.004211881541  , \"κ0\"-> 0.000000005418  , \"mm1\"-> 0.000000000000  , \"mm2\"-> 0.000000000000  , \"mm3\"-> 0.000000000000  , \"T\"->  0.830000000000  , \"B\"-> 8.000000000000  , \"θ\"-> 0.000000000000  |>   , \n\"IDS0387_210910_RAW_cal__sam_\" ->   <| \"ζ\"->  0.013958531253  , \"τ1\"-> 0.040449551738  , \"τS\"-> 0.038075316972  , \"τN\"-> 0.000218997482  , \"τC\"-> 0.005348147372  , \"κ0\"-> 0.000000005866  , \"mm1\"-> 0.000000000000  , \"mm2\"-> 0.000000000000  , \"mm3\"-> 0.000000000000  , \"T\"->  0.830000000000  , \"B\"-> 8.000000000000  , \"θ\"-> 0.000000000000  |>   , \n\"IDS0388_210910_RAW_cal__ref_\" ->   <| \"ζ\"->  0.017074092265  , \"τ1\"-> 0.047215899415  , \"τS\"-> 0.039490388664  , \"τN\"-> 0.000122819272  , \"τC\"-> 0.004722965607  , \"κ0\"-> 0.000000007547  , \"mm1\"-> 0.000000000000  , \"mm2\"-> 0.000000000000  , \"mm3\"-> 0.000000000000  , \"T\"->  1.130000000000  , \"B\"-> 8.000000000000  , \"θ\"-> 0.000000000000  |>   , \n\"IDS0388_210910_RAW_cal__sam_\" ->   <| \"ζ\"->  0.011551866824  , \"τ1\"-> 0.040411227639  , \"τS\"-> 0.048181354691  , \"τN\"-> 0.000103559724  , \"τC\"-> 0.006232382617  , \"κ0\"-> 0.000000008161  , \"mm1\"-> 0.000000000000  , \"mm2\"-> 0.000000000000  , \"mm3\"-> 0.000000000000  , \"T\"->  1.130000000000  , \"B\"-> 8.000000000000  , \"θ\"-> 0.000000000000  |>   , \n\"IDS0389_210910_RAW_cal__ref_\" ->   <| \"ζ\"->  0.017157539727  , \"τ1\"-> 0.046379456311  , \"τS\"-> 0.015264158508  , \"τN\"-> 0.000057006071  , \"τC\"-> 0.004702188691  , \"κ0\"-> 0.000000010470  , \"mm1\"-> 0.000000000000  , \"mm2\"-> 0.000000000000  , \"mm3\"-> 0.000000000000  , \"T\"->  1.520000000000  , \"B\"-> 8.000000000000  , \"θ\"-> 0.000000000000  |>   , \n\"IDS0389_210910_RAW_cal__sam_\" ->   <| \"ζ\"->  0.011148198813  , \"τ1\"-> 0.038849151842  , \"τS\"-> 0.019213865355  , \"τN\"-> 0.000045035153  , \"τC\"-> 0.005536708133  , \"κ0\"-> 0.000000011229  , \"mm1\"-> 0.000000000000  , \"mm2\"-> 0.000000000000  , \"mm3\"-> 0.000000000000  , \"T\"->  1.520000000000  , \"B\"-> 8.000000000000  , \"θ\"-> 0.000000000000  |>   , \n\"IDS0390_210910_RAW_cal__ref_\" ->   <| \"ζ\"->  0.016425367394  , \"τ1\"-> 0.039829137916  , \"τS\"-> 0.010121167967  , \"τN\"-> 0.000033814494  , \"τC\"-> 0.004533563026  , \"κ0\"-> 0.000000013089  , \"mm1\"-> 0.000000000000  , \"mm2\"-> 0.000000000000  , \"mm3\"-> 0.000000000000  , \"T\"->  1.900000000000  , \"B\"-> 8.000000000000  , \"θ\"-> 0.000000000000  |>   , \n\"IDS0390_210910_RAW_cal__sam_\" ->   <| \"ζ\"->  0.010826949430  , \"τ1\"-> 0.038768037521  , \"τS\"-> 0.012925317198  , \"τN\"-> 0.000029157336  , \"τC\"-> 0.005196063884  , \"κ0\"-> 0.000000013864  , \"mm1\"-> 0.000000000000  , \"mm2\"-> 0.000000000000  , \"mm3\"-> 0.000000000000  , \"T\"->  1.900000000000  , \"B\"-> 8.000000000000  , \"θ\"-> 0.000000000000  |>   , \n\"IDS0391_210910_RAW_cal__ref_\" ->   <| \"ζ\"->  0.016160769926  , \"τ1\"-> 0.047360928893  , \"τS\"-> 0.041725389227  , \"τN\"-> 0.000076715950  , \"τC\"-> 0.004871049589  , \"κ0\"-> 0.000000008346  , \"mm1\"-> 0.000000000000  , \"mm2\"-> 0.000000000000  , \"mm3\"-> 0.000000000000  , \"T\"->  1.250000000000  , \"B\"-> 8.000000000000  , \"θ\"-> 0.000000000000  |>   , \n\"IDS0391_210910_RAW_cal__sam_\" ->   <| \"ζ\"->  0.010962610928  , \"τ1\"-> 0.040398807374  , \"τS\"-> 0.051328988590  , \"τN\"-> 0.000070281011  , \"τC\"-> 0.006422533164  , \"κ0\"-> 0.000000008958  , \"mm1\"-> 0.000000000000  , \"mm2\"-> 0.000000000000  , \"mm3\"-> 0.000000000000  , \"T\"->  1.250000000000  , \"B\"-> 8.000000000000  , \"θ\"-> 0.000000000000  |>   , \n\"IDS0392_210910_RAW_cal__ref_\" ->   <| \"ζ\"->  0.016250541117  , \"τ1\"-> 0.047393343666  , \"τS\"-> 0.029998719281  , \"τN\"-> 0.000076850447  , \"τC\"-> 0.004810494325  , \"κ0\"-> 0.000000009475  , \"mm1\"-> 0.000000000000  , \"mm2\"-> 0.000000000000  , \"mm3\"-> 0.000000000000  , \"T\"->  1.390000000000  , \"B\"-> 8.000000000000  , \"θ\"-> 0.000000000000  |>   , \n\"IDS0392_210910_RAW_cal__sam_\" ->   <| \"ζ\"->  0.010962610928  , \"τ1\"-> 0.040398807374  , \"τS\"-> 0.051328988590  , \"τN\"-> 0.000070281011  , \"τC\"-> 0.006422533164  , \"κ0\"-> 0.000000008958  , \"mm1\"-> 0.000000000000  , \"mm2\"-> 0.000000000000  , \"mm3\"-> 0.000000000000  , \"T\"->  1.390000000000  , \"B\"-> 8.000000000000  , \"θ\"-> 0.000000000000  |>   , \n\"IDS0393_210910_RAW_cal__ref_\" ->   <| \"ζ\"->  0.015227705493  , \"τ1\"-> 0.038797003927  , \"τS\"-> 0.007286355621  , \"τN\"-> 0.000013994204  , \"τC\"-> 0.003959851165  , \"κ0\"-> 0.000000023455  , \"mm1\"-> 0.000000000000  , \"mm2\"-> 0.000000000000  , \"mm3\"-> 0.000000000000  , \"T\"->  3.110000000000  , \"B\"-> 8.000000000000  , \"θ\"-> 0.000000000000  |>   , \n\"IDS0393_210910_RAW_cal__sam_\" ->   <| \"ζ\"->  0.010962610928  , \"τ1\"-> 0.040398807374  , \"τS\"-> 0.051328988590  , \"τN\"-> 0.000070281011  , \"τC\"-> 0.006422533164  , \"κ0\"-> 0.000000008958  , \"mm1\"-> 0.000000000000  , \"mm2\"-> 0.000000000000  , \"mm3\"-> 0.000000000000  , \"T\"->  3.110000000000  , \"B\"-> 8.000000000000  , \"θ\"-> 0.000000000000  |>   , \n\"IDS0394_210910_RAW_cal__ref_\" ->   <| \"ζ\"->  0.018884017265  , \"τ1\"-> 0.038756536887  , \"τS\"-> 0.005123025136  , \"τN\"-> 0.000004793994  , \"τC\"-> 0.002621800478  , \"κ0\"-> 0.000000058143  , \"mm1\"-> 0.000000000000  , \"mm2\"-> 0.000000000000  , \"mm3\"-> 0.000000000000  , \"T\"->  5.750000000000  , \"B\"-> 8.000000000000  , \"θ\"-> 0.000000000000  |>   , \n\"IDS0394_210910_RAW_cal__sam_\" ->   <| \"ζ\"->  0.010962610928  , \"τ1\"-> 0.040398807374  , \"τS\"-> 0.051328988590  , \"τN\"-> 0.000070281011  , \"τC\"-> 0.006422533164  , \"κ0\"-> 0.000000008958  , \"mm1\"-> 0.000000000000  , \"mm2\"-> 0.000000000000  , \"mm3\"-> 0.000000000000  , \"T\"->  5.750000000000  , \"B\"-> 8.000000000000  , \"θ\"-> 0.000000000000  |>   , \n\"IDS0395_210910_RAW_cal__ref_\" ->   <| \"ζ\"->  0.016101273075  , \"τ1\"-> 0.047373144247  , \"τS\"-> 0.040453117489  , \"τN\"-> 0.000076678480  , \"τC\"-> 0.005036745304  , \"κ0\"-> 0.000000008627  , \"mm1\"-> 0.000000000000  , \"mm2\"-> 0.000000000000  , \"mm3\"-> 0.000000000000  , \"T\"->  1.310000000000  , \"B\"-> 8.000000000000  , \"θ\"-> 0.000000000000  |>   , \n\"IDS0395_210910_RAW_cal__sam_\" ->   <| \"ζ\"->  0.010962610928  , \"τ1\"-> 0.040398807374  , \"τS\"-> 0.051328988590  , \"τN\"-> 0.000070281011  , \"τC\"-> 0.006422533164  , \"κ0\"-> 0.000000008958  , \"mm1\"-> 0.000000000000  , \"mm2\"-> 0.000000000000  , \"mm3\"-> 0.000000000000  , \"T\"->  1.310000000000  , \"B\"-> 8.000000000000  , \"θ\"-> 0.000000000000  |>   , \n"
